vi "KelvinToFar.vi"(11 "Кельвин":dbl) -> (3 "Фаренгейт":dbl)   [LabVIEW 2017]
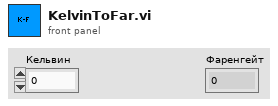
[diagram p1: front panel]
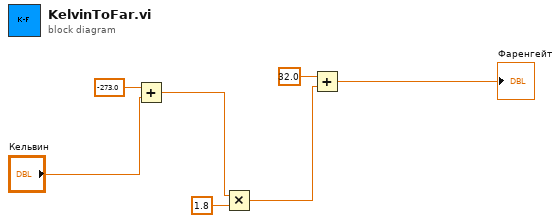
[diagram p0: block diagram]
diagram:
  n1 = Add(x=-273.0, y="Кельвин") -> (x+y=w4:dbl)
  n2 = Multiply(x=w4, y=1.8) -> (x*y=w3:dbl)
  n3 = Add(x=32.0, y=w3) -> (x+y=→"Фаренгейт":dbl)
